vi "AttackHim.vi"(8 "error in (no error)":errorcluster, 9 "Cube":i32, 10 "Rival":refnum<class "Peasant.lvclass">, 11 "Knight in":refnum<class "Knight.lvclass">) -> (0 "error out":errorcluster, 1 "CurrentAttack":i32, 2 "Rival out":refnum<class "Peasant.lvclass">, 3 "Knight out":refnum<class "Knight.lvclass">)   [LabVIEW 2021, in "Knight.lvclass"]
uses:
  Knight.lvclass
  W:/School/AnimoProgramovani2/2023/LabVIEW/Arena/Peasant/Peasant.lvclass
  Peasant/Peasant.lvclass
  Peasant/Peasant.lvclass/Peasant.ctl
  Peasant/Read Peasant Attributes.vi
  Peasant/Write Peasant Attributes.vi
  Knight.lvclass/Knight.ctl
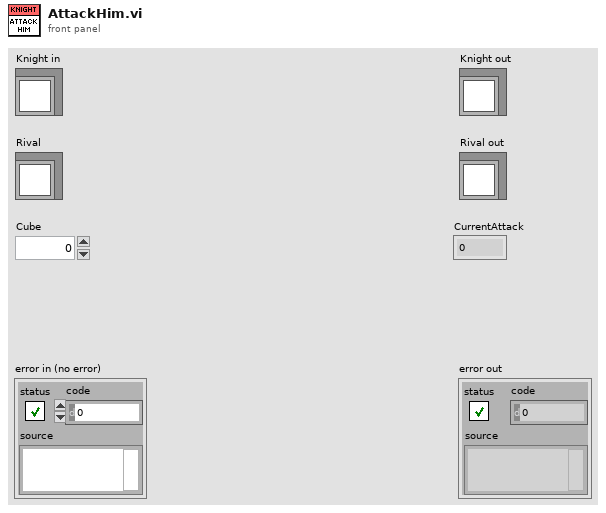
[diagram p1: front panel]
types:
  T1 = typedef "Peasant.lvclass/PeasantAttributes.ctl" = cluster{"Health":i32, "Stamina":i32, "Attack":i32, "Defense":i32, "Sing":i32}
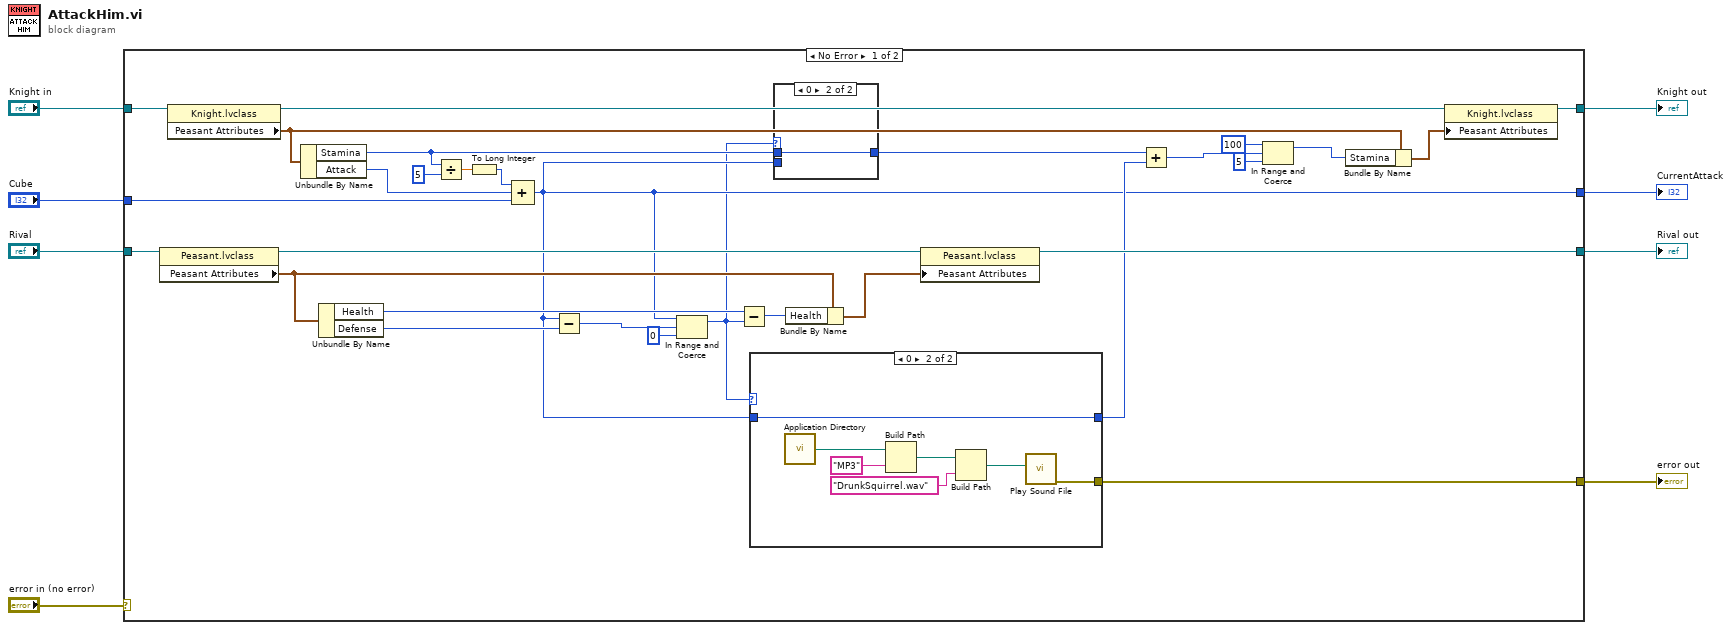
[diagram p0: block diagram]
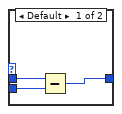
[diagram p2: hidden frame]
diagram:
  n1 = case shown="No Error" "error in (no error)" {
    selector: "error in (no error)" -> [_ w52]
    tunnel: [w23 w52] -> w2
    tunnel: [w24 w51] -> w4
    tunnel: "Knight in" -> [w38 w51]
    tunnel: "Rival" -> [w37 w50]
    tunnel: "Cube" -> [w16 _]
    tunnel: [w31 w50] -> w1
    tunnel: [w11 _] -> w3
    frame No Error {
      n2 = property class="Peasant.lvclass"(reference=w37) -> (reference out=w33:refnum<class "Peasant.lvclass">, "Peasant Attributes"=w35:T1)  [unwired: 1 in, 1 out]
      n3 = property class="Knight.lvclass"(reference=w38) -> (reference out=w27:refnum<class "Knight.lvclass">, "Peasant Attributes"=w26:T1)  [unwired: 1 in, 1 out]
      n4 = Unbundle By Name(w26) -> ("Stamina"=w15:i32, "Attack"=w17:i32)
      n5 = Unbundle By Name(w35) -> ("Health"=w36:i32, "Defense"=w30:i32)
      n6 = Divide(x=w15, y=5) -> (x/y=w13:dbl)
      n7 = To Long Integer(number=w13) -> (32bit integer=w12:i32)
      n8 = Compound Arithmetic op=ADD(w12, w17, w16) -> (w11:i32)
      n9 = Subtract(x=w11, y=w30) -> (x-y=w28:i32)
      n10 = In Range and Coerce(upper limit=w11, x=w28, lower limit=0) -> (coerced(x)=w9:i32)  [unwired: 1 out]
      n11 = Subtract(x=w36, y=w9) -> (x-y=w34:i32)
      n12 = case shown="0" w9 {
        tunnel: [_ w44] -> w23
        tunnel: w11 -> [_ w43]
        tunnel: [_ w43] -> w21
        frame Default {
        }
        frame 0 {
          n13 = call <vilib>:"Application Directory.vi"() -> ("Application Directory"=w49:path)
          n14 = Build Path(base path=w49, name or relative path="MP3") -> (appended path=w47:path)
          n15 = Build Path(base path=w47, name or relative path="DrunkSquirrel.wav") -> (appended path=w45:path)
          n16 = call <vilib>:"Play Sound File.vi"("path"=w45) -> ("error out"=w44:errorcluster)  [unwired: 9 in, 1 out]
        }
      }
      n17 = case shown="0" w9 {
        tunnel: [w41 w42] -> w22
        tunnel: w15 -> [w40 w42]
        tunnel: w11 -> [w39 _]
        frame Default {
          n18 = Subtract(x=w40, y=w39) -> (x-y=w41:i32)
        }
        frame 0 {
        }
      }
      n19 = Bundle By Name(cluster=w35, "Health"=w34) -> (w32:T1)
      n20 = property class="Peasant.lvclass"(reference=w33, "Peasant Attributes"=w32) -> (reference out=w31:refnum<class "Peasant.lvclass">)  [unwired: 1 in, 1 out]
      n21 = Add(x=w22, y=w21) -> (x+y=w20:i32)
      n22 = In Range and Coerce(upper limit=100, x=w20, lower limit=5) -> (coerced(x)=w18:i32)  [unwired: 1 out]
      n23 = Bundle By Name(cluster=w26, "Stamina"=w18) -> (w25:T1)
      n24 = property class="Knight.lvclass"(reference=w27, "Peasant Attributes"=w25) -> (reference out=w24:refnum<class "Knight.lvclass">)  [unwired: 1 in, 1 out]
    }
    frame Error {
    }
  }
  "error out" <- w2
  "Knight out" <- w4
  "Rival out" <- w1
  "CurrentAttack" <- w3
